vi "ReadSF_9002.vi"(0 "connection ID in":refnum<k5>, 1 "error in":errorcluster, 2 "enabled":bool, 3 "bytes to read":i32, 4 "timeout (optional)":dbl=inf, 5 "header size":i32) -> (6 "connection ID out":refnum<k5>, 7 "string":string, 8 "error out":errorcluster)   [LabVIEW 2011]
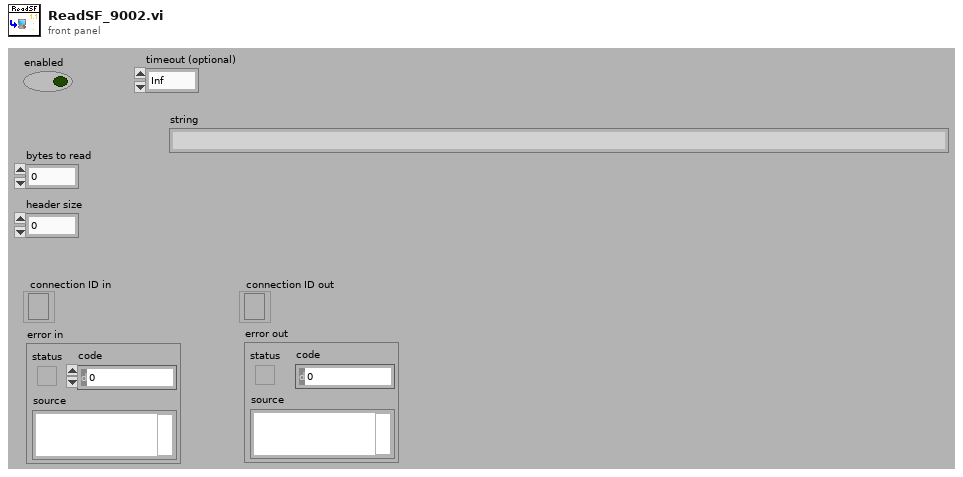
[diagram p1: front panel]
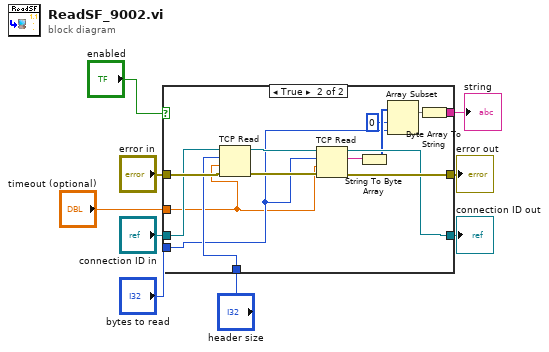
[diagram p0: block diagram]
diagram:
  n1 = case shown="True" "enabled" {
    tunnel: [w11 w25] -> w9
    tunnel: "error in" -> [w11 w19]
    tunnel: "connection ID in" -> [w10 w16]
    tunnel: [w10 w24] -> w5
    tunnel: "bytes to read" -> [_ w13]
    tunnel: "header size" -> [_ w15]
    tunnel: [_ w20] -> w2
    tunnel: "timeout (optional)" -> [_ w12]
    frame False {
    }
    frame True {
      n2 = TCP Read(connection ID=w16, bytes to read=w15, error in (no error)=w19, 9:w12) -> (connection ID out=w17:refnum<k5>, error out=w18:errorcluster)  [unwired: 1 in, 1 out]
      n3 = TCP Read(connection ID=w17, bytes to read=w13, error in (no error)=w18, 9:w12) -> (connection ID out=w24:refnum<k5>, data out=w23:string, error out=w25:errorcluster)  [unwired: 1 in]
      n4 = String To Byte Array(string=w23) -> (unsigned byte array=w22:u8[])
      n5 = Array Subset(array=w22, index=0, length=w13) -> (w21:u8[])
      n6 = Byte Array To String(unsigned byte array=w21) -> (string=w20:string)
    }
  }
  "error out" <- w9
  "connection ID out" <- w5
  "string" <- w2
